vi "graph_change_point_finder_fury.vi"(8 "Scan length":i32=30, 11 "subarray 2":dbl[](array[numeric])) -> (3 "Trace Change point":i32)   [LabVIEW 2015]
uses:
  <vilib>/Analysis/baseanly.llb/Mean (DBL).vi
  <vilib>/Analysis/NI_AALBase.lvlib
panel:
  in  "Data offset":i32=10
  out "Waveform Graph":dbl[][](graph)
  out "size(s)":i32
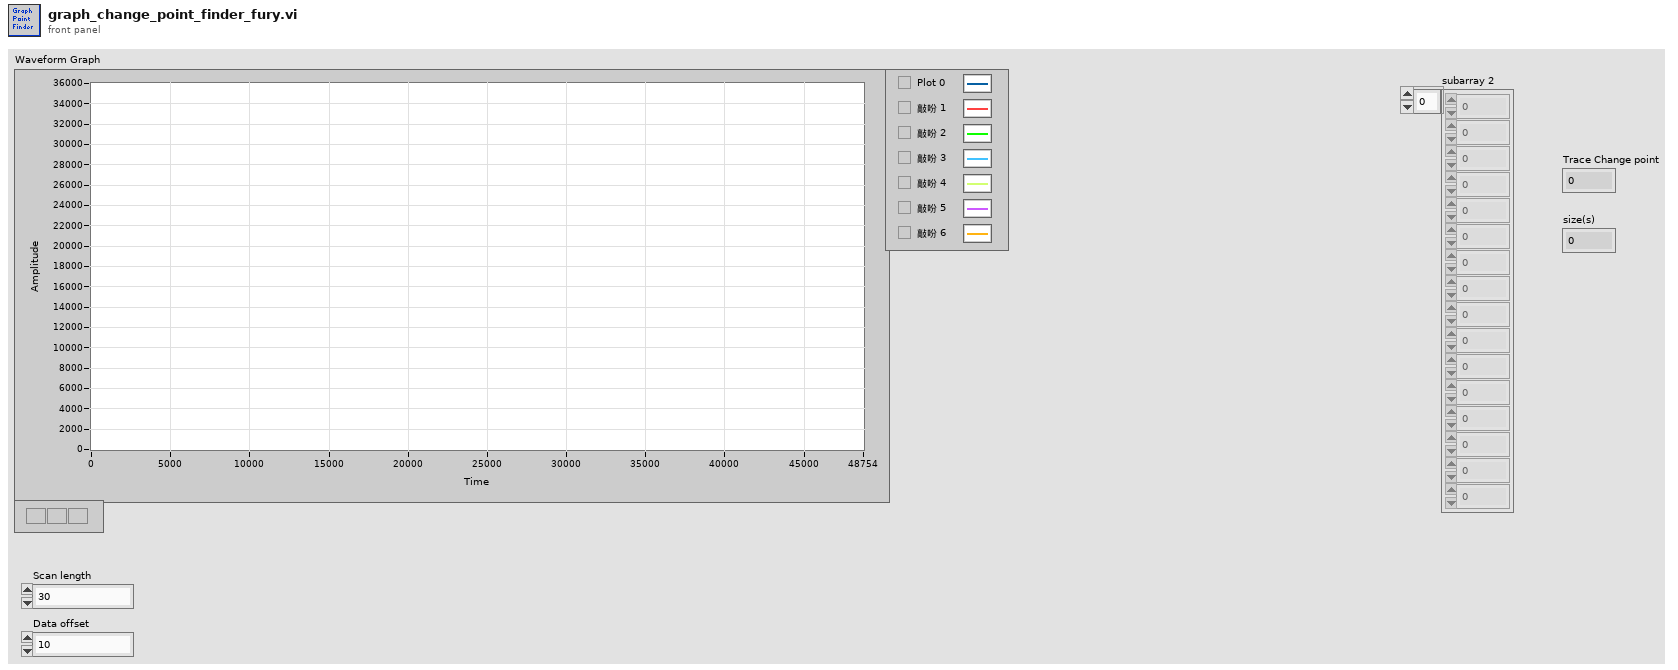
[diagram p1: front panel]
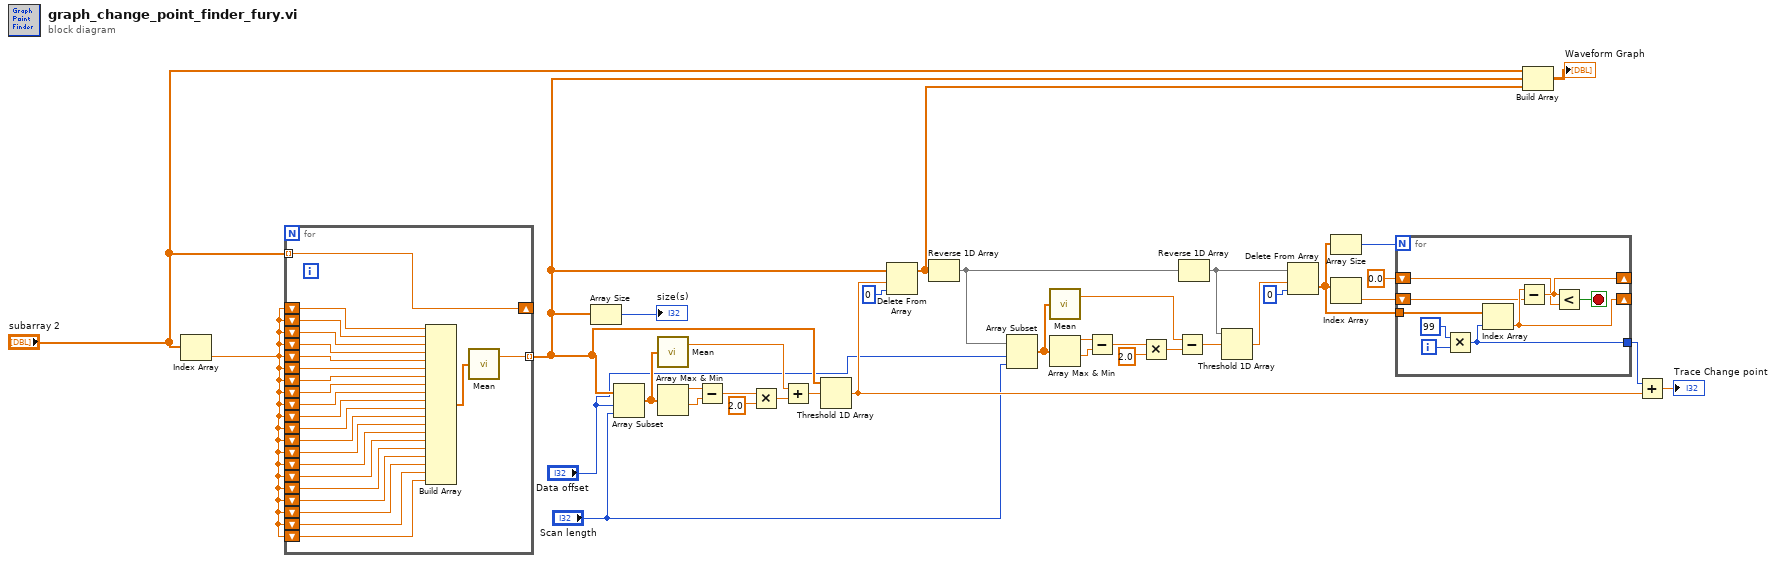
[diagram p0: block diagram]
diagram:
  n1 = Index Array(array="subarray 2") -> (element=w13:dbl)  [unwired: 1 in]
  n2 = for {
    tunnel: "subarray 2" -> [w59] mode=indexing
    shift-right: [w59] -> _
    shift-left: w13 -> [w54]
    shift-left: w13 -> [w57]
    shift-left: w13 -> [w58]
    shift-left: w13 -> [w56]
    shift-left: w13 -> [w55]
    tunnel: [w52] -> w12 mode=indexing
    shift-left: w13 -> [w47]
    shift-left: w13 -> [w48]
    shift-left: w13 -> [w49]
    shift-left: w13 -> [w50]
    shift-left: w13 -> [w51]
    shift-left: w13 -> [w46]
    shift-left: w13 -> [w45]
    shift-left: w13 -> [w44]
    shift-left: w13 -> [w43]
    shift-left: w13 -> [w42]
    shift-left: w13 -> [w41]
    shift-left: w13 -> [w40]
    shift-left: w13 -> [w39]
    shift-left: w13 -> [w38]
    shift-left: w13 -> [w37]
    n3 = Build Array(w51, w50, w49, w48, w47, w54, w57, w58, w56, w55, w46, w45, w44, w43, w42, w41, w40, w39, w38, w37) -> (w53:dbl[])
    n4 = call-poly <vilib>:"Mean.vi"("X"=w53) -> ("mean"=w52:dbl)  [unwired: 1 out]
  }
  n5 = Array Size(array=w12) -> (size(s)=→"size(s)":i32)
  n6 = Array Subset(array=w12, index="Data offset", length="Scan length") -> (w35:dbl[])
  n7 = call-poly <vilib>:"Mean.vi"("X"=w35) -> ("mean"=w34:dbl)  [unwired: 1 out]
  n8 = Array Max & Min(array=w35) -> (max value=w9:dbl, min value=w8:dbl)  [unwired: 2 out]
  n9 = Subtract(x=w9, y=w8) -> (x-y=w7:dbl)
  n10 = Multiply(x=w7, y=2.0) -> (x*y=w6:dbl)
  n11 = Add(x=w34, y=w6) -> (x+y=w33:dbl)
  n12 = Threshold 1D Array(2:w33, 3:w12) -> (0:w15:dbl)  [unwired: 1 in]
  n13 = Delete From Array(array=w12, length=w15, index=0) -> (array with subset deleted=w10:dbl[])  [unwired: 1 out]
  n14 = Reverse 1D Array(array=w10) -> (reversed array=w21:dbl[])
  n15 = Array Subset(array=w21, index="Data offset", length="Scan length") -> (w24:dbl[])
  n16 = call-poly <vilib>:"Mean.vi"("X"=w24) -> ("mean"=w30:dbl)  [unwired: 1 out]
  n17 = Array Max & Min(array=w24) -> (max value=w25:dbl, min value=w26:dbl)  [unwired: 2 out]
  n18 = Subtract(x=w25, y=w26) -> (x-y=w27:dbl)
  n19 = Multiply(x=w27, y=2.0) -> (x*y=w29:dbl)
  n20 = Subtract(x=w30, y=w29) -> (x-y=w31:dbl)
  n21 = Reverse 1D Array(array=w21) -> (reversed array=w20:dbl[])
  n22 = Threshold 1D Array(2:w31, 3:w20) -> (0:w22:dbl)  [unwired: 1 in]
  n23 = Delete From Array(array=w20, length=w22, index=0) -> (deleted portion=w5:dbl[])  [unwired: 1 out]
  n24 = Array Size(array=w5) -> (size(s)=w17:i32)
  n25 = Index Array(array=w5) -> (element=w19:dbl)  [unwired: 1 in]
  n26 = for {
    N: w17 -> [_]
    tunnel: w5 -> [w68]
    shift-right: [w65] -> _
    shift-left: w19 -> [w64]
    shift-right: [w63] -> _
    shift-left: 0.0 -> [w62]
    tunnel: [w60] -> w16
    i -> [w67]
    stop <- w61 stop-if-true
    n27 = Multiply(x=99, y=w67) -> (x*y=w60:i32)
    n28 = Index Array(array=w68, index=w60) -> (element=w65:dbl)
    n29 = Subtract(x=w65, y=w64) -> (x-y=w63:dbl)
    n30 = Less?(x=w63, y=w62) -> (x < y?=w61:bool)
  }
  n31 = Build Array("subarray 2", w12, w10) -> (→"Waveform Graph":dbl[][])
  n32 = Add(x=w16, y=w15) -> (x+y=→"Trace Change point":dbl)
